vi "Check.vi"(6 "Peripherals in":T1, 8 "error in (no error)":errorcluster) -> (0 "error out":errorcluster, 1 "motor ok?":bool[](array[boolean]), 2 "auto off?":bool, 4 "Peripherals out":T1, 5 "auto off resp":string)   [LabVIEW 2014, in "AISAS Mech.lvclass"]
uses:
  AISAS Mech.lvclass
  Controls/peripherals.ctl
  AISAS Mech.lvclass/AISAS Mech.ctl
  motor/AISAS motor.lvclass
panel:
  # "rot\ndiff\nfocus"
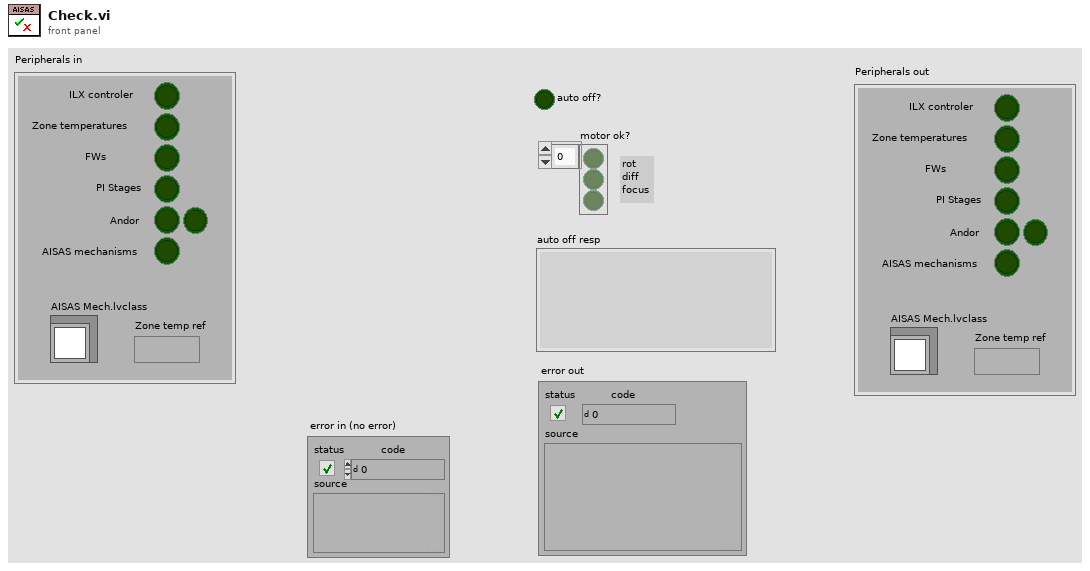
[diagram p1: front panel]
types:
  T1 = typedef "peripherals.ctl" = cluster{"ILX controler":bool, "Zone temperatures":bool, "Andor":bool, "Andor 2":bool, "PI Stages":bool, "AISAS mechanisms":bool, "AISAS Mech.lvclass":refnum<class "AISAS Mech.lvclass">, "Zone temp ref":variant, "FWs":bool}
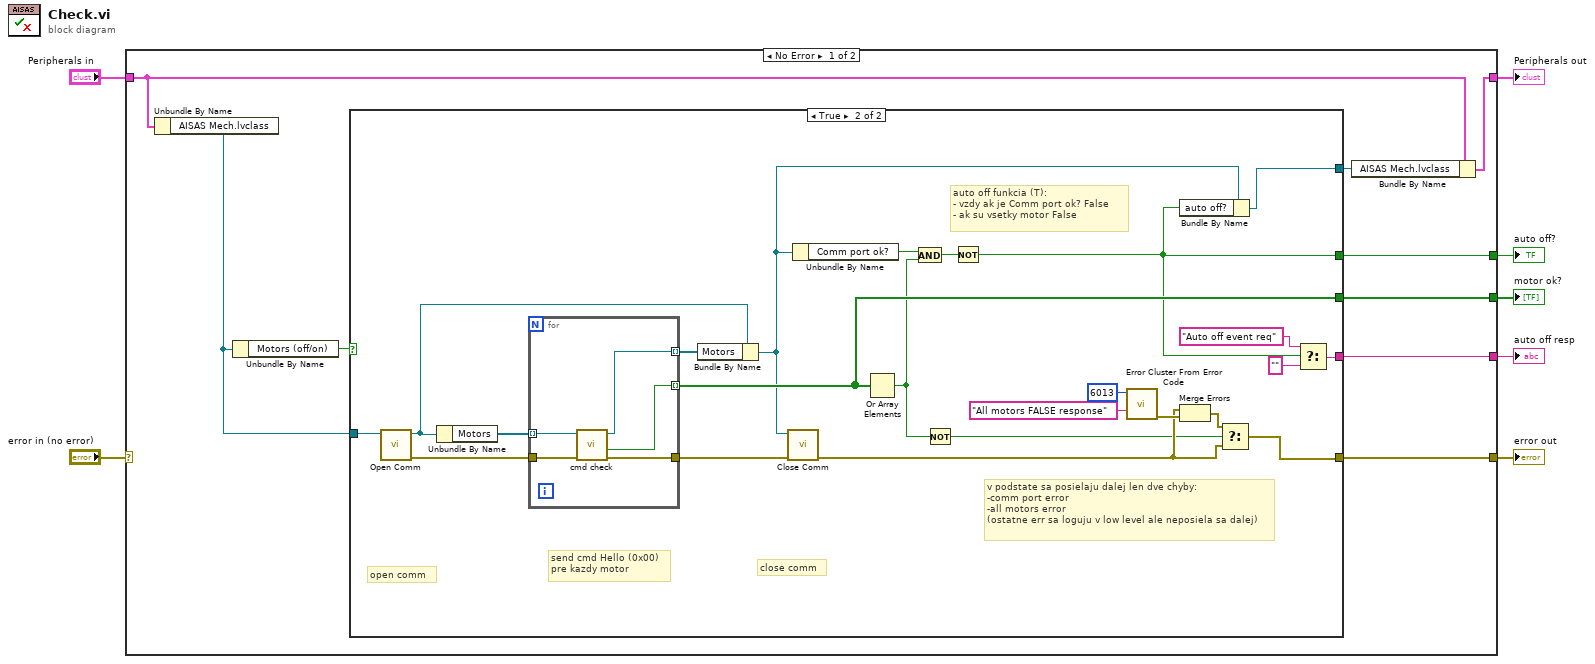
[diagram p0: block diagram]
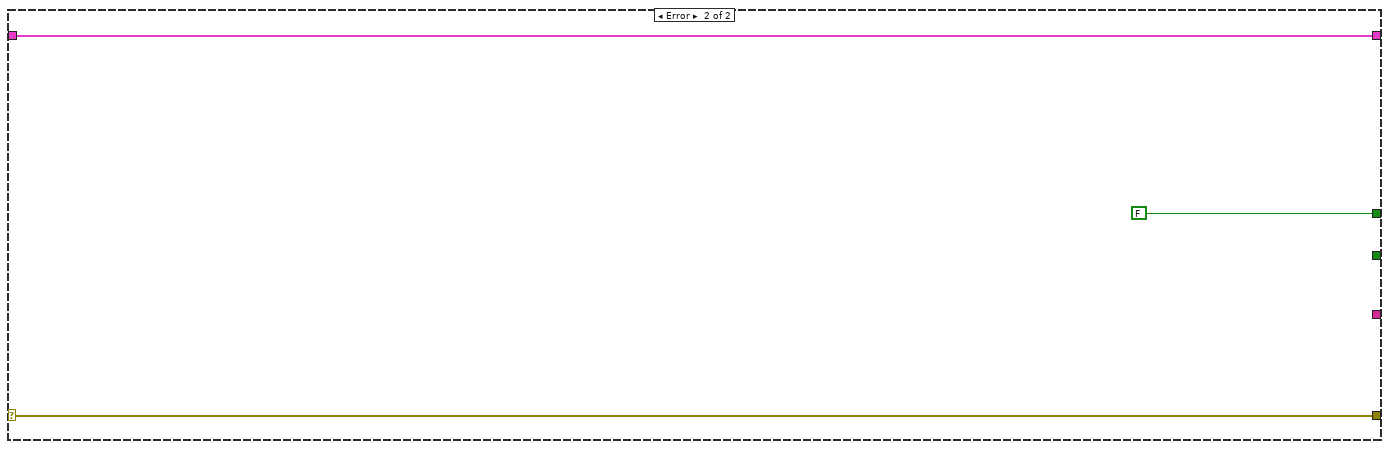
[diagram p3: hidden frame]
diagram:
  n1 = case shown="No Error" "error in (no error)" {
    selector: "error in (no error)" -> [_ w49]
    tunnel: [w16 _] -> w7
    tunnel: [w15 w49] -> w6
    tunnel: [w14 _] -> w4
    tunnel: [w13 FALSE] -> w3
    tunnel: "Peripherals in" -> [w9 w47]
    tunnel: [w8 w47] -> w1
    frame No Error {
      n2 = Unbundle By Name(w9) -> ("AISAS Mech.lvclass"=w11:refnum<class "AISAS Mech.lvclass">)
      n3 = Unbundle By Name(w11) -> ("Motors (off/on)"=w12:bool)
      n4 = case shown="True" w12 {
        selector: w12 -> [w17 _]
        tunnel: [_ w39] -> w16
        tunnel: [_ w24] -> w15
        tunnel: [_ w33] -> w14
        tunnel: w11 -> [w18 w38]
        tunnel: [w18 w40] -> w10
        tunnel: [w17 w34] -> w13
        frame False {
        }
        frame True {
          # "v podstate sa posielaju dalej len dve chyby:\n-comm port error\n-all motors error\n(ostatne err sa loguju v low level ale neposiela sa dalej)"
          # "auto off funkcia (T):\n- vzdy ak je Comm port ok? False\n- ak su vsetky motor False"
          # "close comm"
          # "send cmd Hello (0x00)\npre kazdy motor"
          # "open comm"
          n5 = call "Open Comm.vi"("AISAS Mech in"=w38) -> ("error out"=w41:errorcluster, "AISAS Mech out"=w36:refnum<class "AISAS Mech.lvclass">)  [unwired: 8 in, 1 out]
          n6 = Unbundle By Name(w36) -> ("Motors"=w21:refnum<class "AISAS motor.lvclass">[])
          n7 = for {
            tunnel: [w45] -> w39 mode=indexing
            tunnel: w41 -> [w46]
            tunnel: [w44] -> w23
            tunnel: w21 -> [w43] mode=indexing
            tunnel: [w42] -> w20 mode=indexing
            n8 = call "cmd check.vi"("error in (no error)"=w46, "motor in"=w43) -> ("error out"=w44:errorcluster, "Motor Ok?"=w45:bool, "motor out"=w42:refnum<class "AISAS motor.lvclass">)  [unwired: 7 in]
          }
          n9 = Bundle By Name(cluster=w36, "Motors"=w20) -> (w19:refnum<class "AISAS Mech.lvclass">)
          n10 = call "Close Comm.vi"("error in (no error)"=w23, "AISAS Mech"=w19) -> ("error out"=w25:errorcluster)  [unwired: 9 in]
          n11 = Unbundle By Name(w19) -> ("Comm port ok?"=w37:bool)
          n12 = Or Array Elements(Boolean array=w39) -> (logical OR=w26:bool)
          n13 = And(x=w37, y=w26) -> (x .and. y?=w35:bool)
          n14 = Not(x=w26) -> (.not. x?=w22:bool)
          n15 = Not(x=w35) -> (.not. x?=w34:bool)
          n16 = call <vilib>:"Error Cluster From Error Code.vi"("error message (\"\")"="All motors FALSE response" ("error message (\"\")"), "error code (0)"=6013) -> ("error out"=w28:errorcluster)  [unwired: 7 in]
          n17 = Bundle By Name(cluster=w19, "auto off?"=w34) -> (w40:refnum<class "AISAS Mech.lvclass">)
          n18 = Merge Errors(w25, w28) -> (w27:errorcluster)
          n19 = Select(t=w27, s=w22, f=w25) -> (s? t:f=w24:errorcluster)
          n20 = Select(t="Auto off event req", s=w34, f="") -> (s? t:f=w33:string)
        }
      }
      n21 = Bundle By Name(cluster=w9, "AISAS Mech.lvclass"=w10) -> (w8:T1)
    }
    frame Error {
    }
  }
  "motor ok?" <- w7
  "error out" <- w6
  "auto off resp" <- w4
  "auto off?" <- w3
  "Peripherals out" <- w1
